vi "FitCoefficientsCalculation.vi"(6 "Iteration > 1/200*arraySize":bool, 8 "Iteration":i32, 9 "fitCoeffMin":i32, 10 "Numeric 4":i16, 11 "Pi/ArraySize":dbl) -> (2 "fitCoefficients.a-b":dbl, 3 "fitCoefficients.Factor":i16)   [LabVIEW 2016]
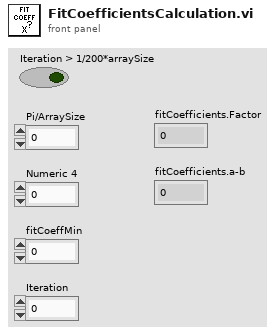
[diagram p1: front panel]
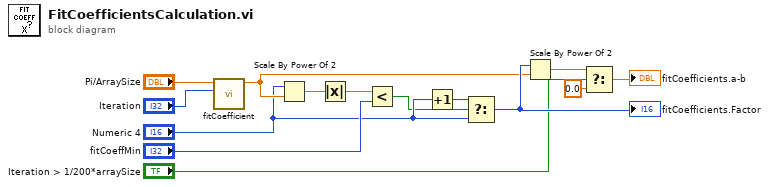
[diagram p0: block diagram]
diagram:
  n1 = call "fitCoefficient.vi"("n"="Iteration", "a"="Pi/ArraySize") -> ("c"=w6:dbl)  [unwired: 8 in, 1 out]
  n2 = Scale By Power Of 2(n="Numeric 4", x=w6) -> (x*2^n=w1:dbl)
  n3 = Absolute Value(x=w1) -> (abs(x)=w5:dbl)
  n4 = Less?(x=w5, y="fitCoeffMin") -> (x < y?=w2:bool)
  n5 = Increment(x="Numeric 4") -> (x+1=w4:i16)
  n6 = Select(t=w4, s=w2, f="Numeric 4") -> (s? t:f=w14:i16)
  "fitCoefficients.Factor" <- w14
  n7 = Scale By Power Of 2(n=w14, x=w6) -> (x*2^n=w7:dbl)
  n8 = Select(t=w7, s="Iteration > 1/200*arraySize", f=0.0) -> (s? t:f=→"fitCoefficients.a-b":dbl)
